vi "Camera.vi"() -> ()   [LabVIEW 2016]
uses:
  <vilib>/rvi/Emulation/niFpgaGetClockAttributes.vi
  <vilib>/rvi/Emulation/niFpgaSctlEmulationGetInTimedLoop.vi
  <vilib>/rvi/Emulation/niFpgaEmulationReportErrorSimple.vi
  <vilib>/rvi/eio/common/nirviEmuTemplateMethod_errors.vi
  <vilib>/rvi/Emulation/niFpgaCriticalErrorInLSC.vi
  <vilib>/eio/EIONode/EIONode.xnode
panel:
  in  "Fly View Frame Rate = R 2":i16=10
  in  "Tlow = t":i16=9
  in  "Arena View Frame Rate = R":i16=200
  out "Camera flash time":i16
  in  "Camera flash time t":i16
  in  "Flash":bool
  # "** Frequency  = 1 / (Fly View R * 0.0001)   i.e R = 10, Frequency = 1000Hz"
  # "**T period = R*100µs,      T low = t*100 µs"
  # "** Frequency  = 1 / (R * 0.0001)   i.e R = 100, Frequency = 100Hz"
  # "** Trigger the fluorenscence camera (Arena View R - x ) *100 microseconds earlier\n      i.e Arena View R = 100, x = 98,\n           offset x = (100 - 98) * 100 µs = 200 µs"
  # "** Camera flash time is set to be the time for triggering the flash at the end of every video.\n** The unit is second."
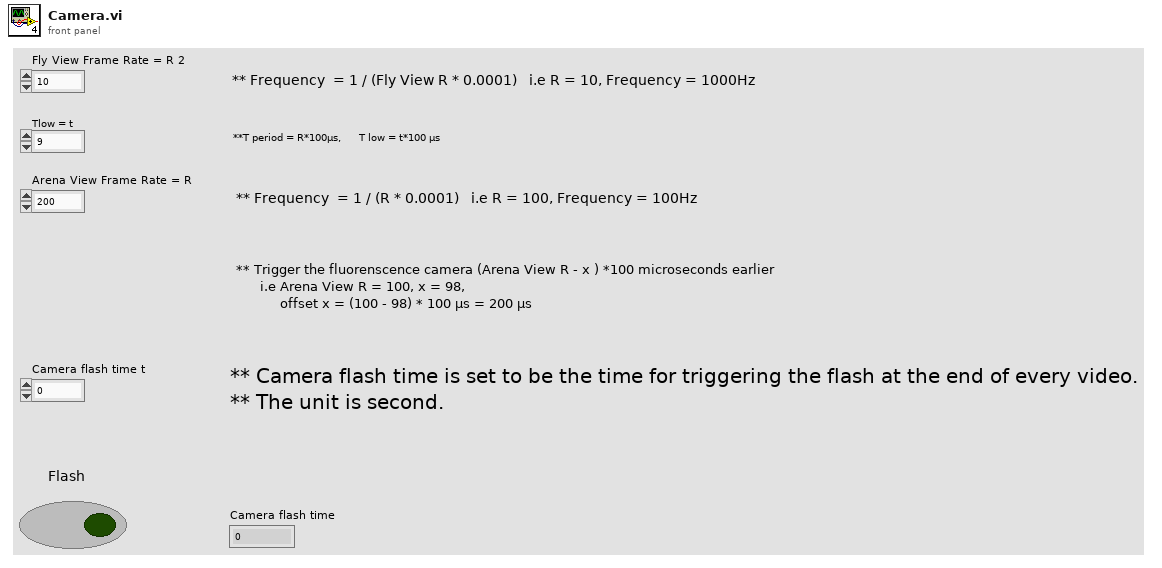
[diagram p1: front panel]
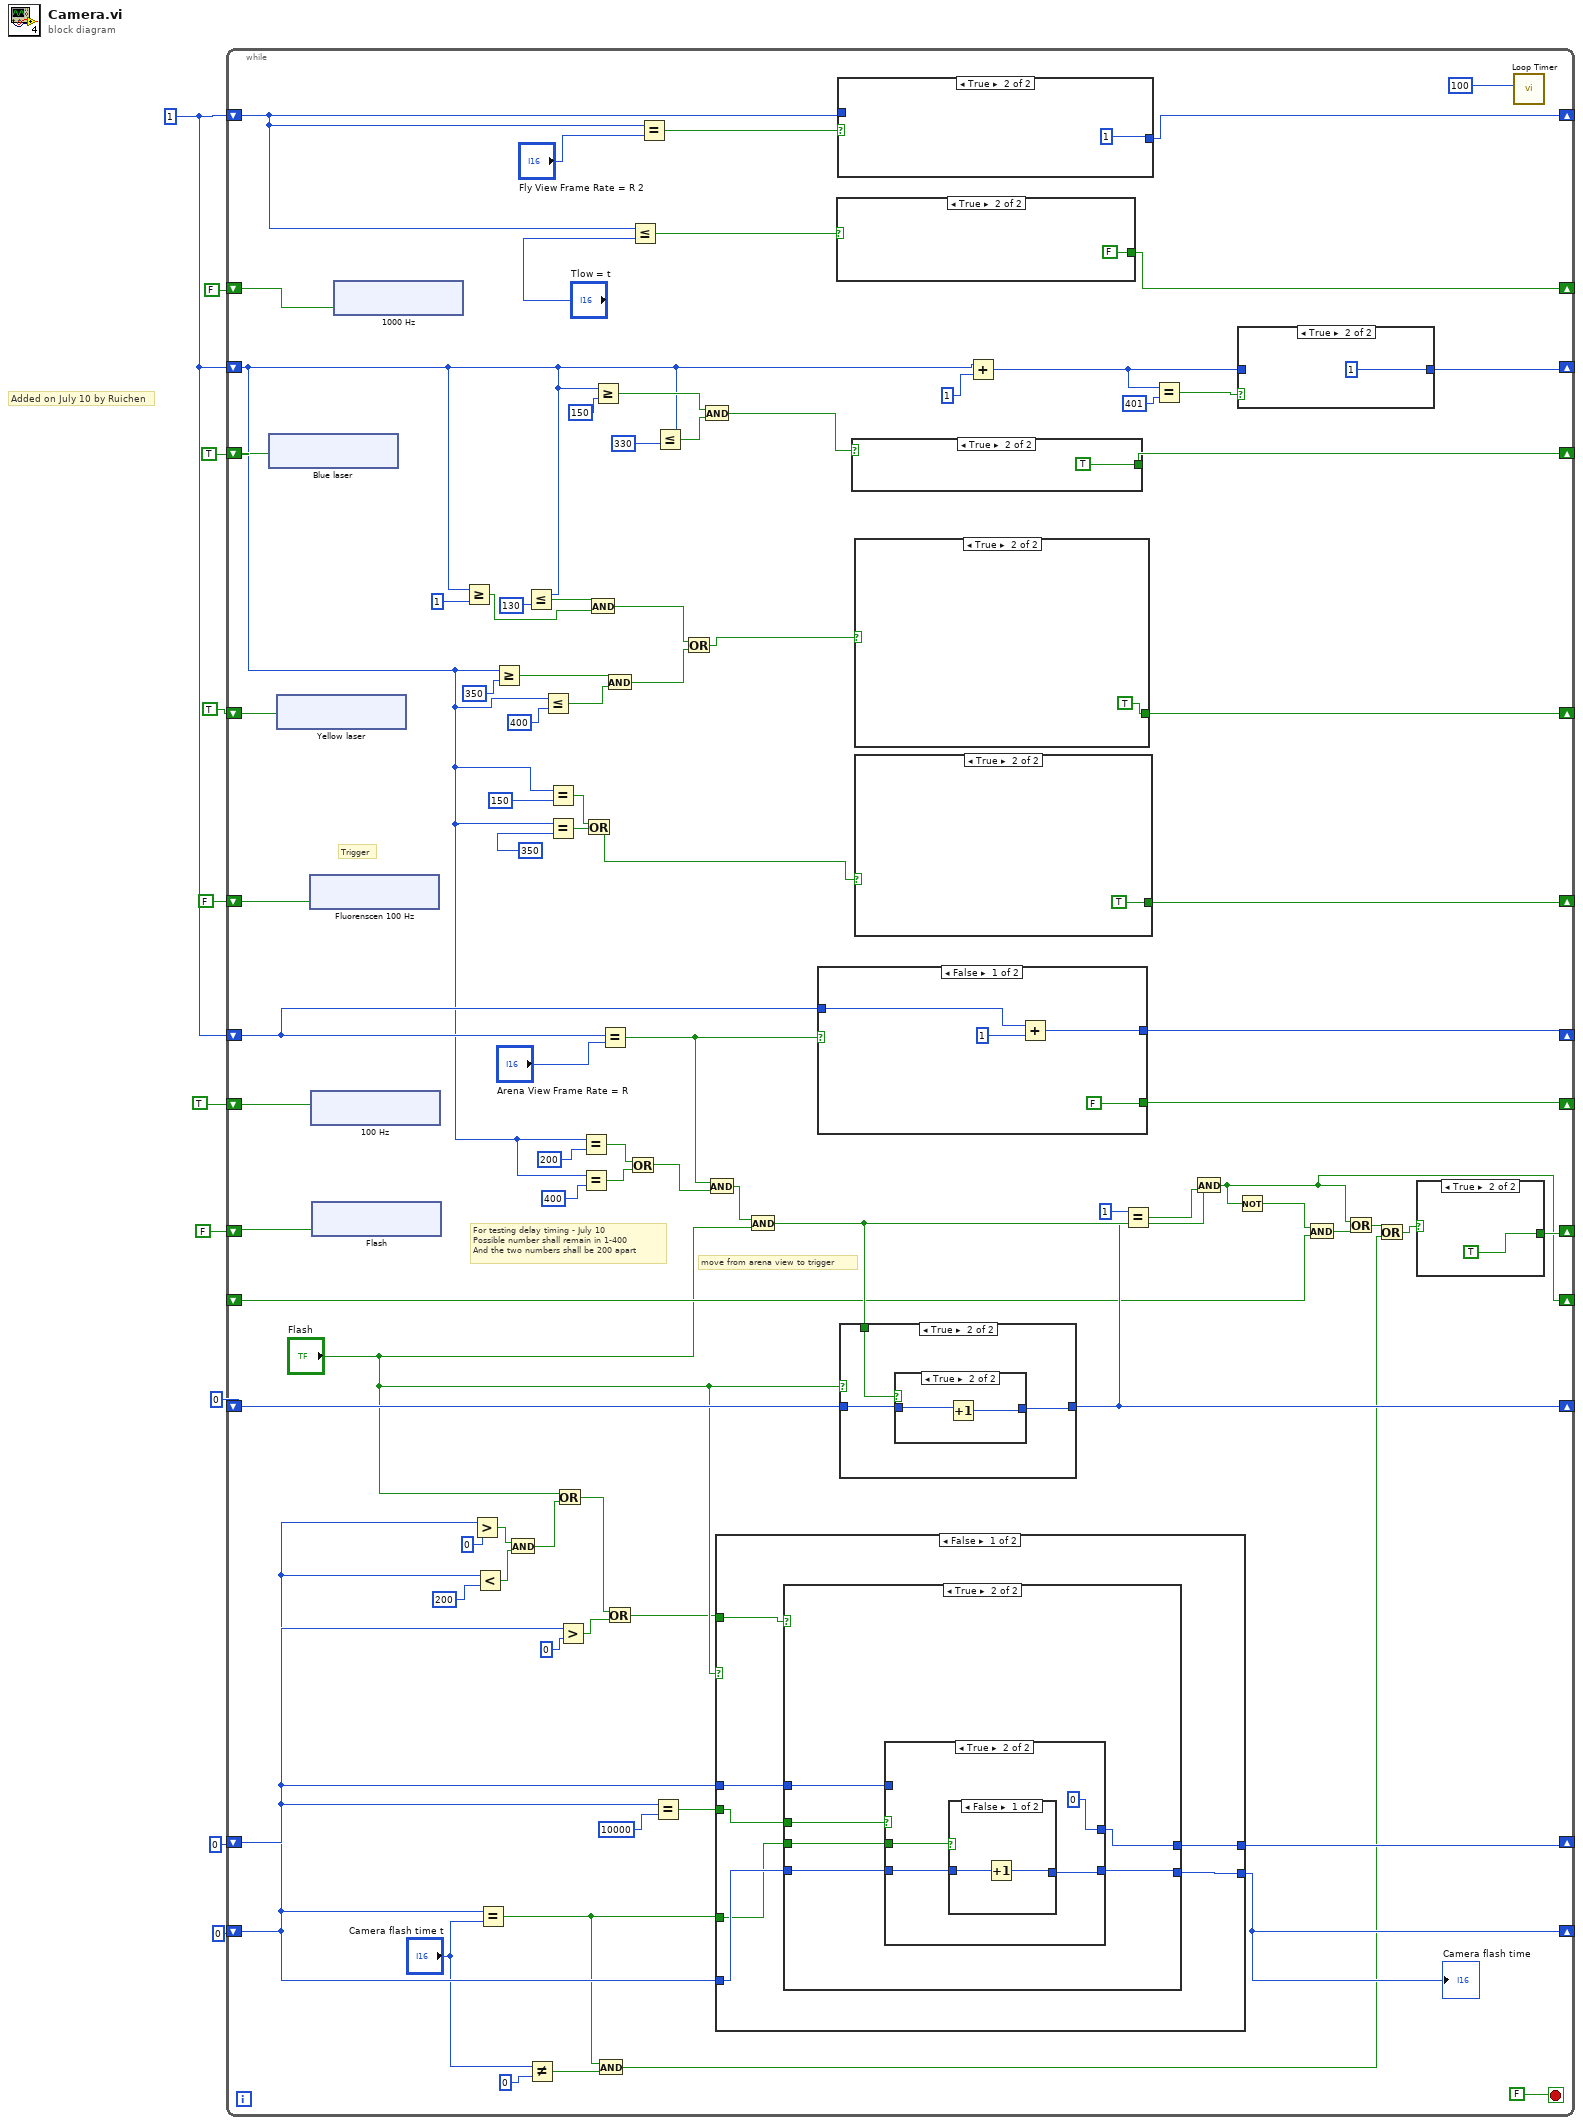
[diagram p0: block diagram]
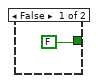
[diagram p2: hidden frame]
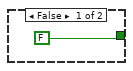
[diagram p4: hidden frame]
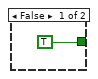
[diagram p5: hidden frame]
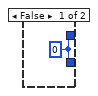
[diagram p6: hidden frame]
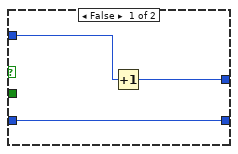
[diagram p7: hidden frame]
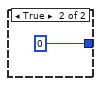
[diagram p8: hidden frame]
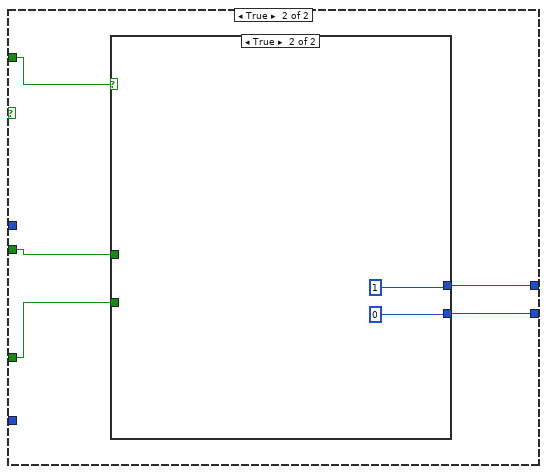
[diagram p9: hidden frame]
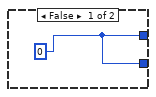
[diagram p10: hidden frame]
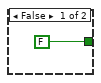
[diagram p11: hidden frame]
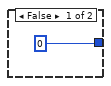
[diagram p12: hidden frame]
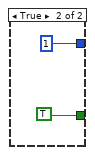
[diagram p14: hidden frame]
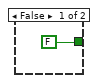
[diagram p15: hidden frame]
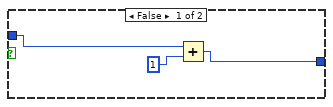
[diagram p16: hidden frame]
diagram:
  w1 = i16 1
  # "Added on July 10 by Ruichen"
  n1 = while {
    shift-right: [w54] -> _
    shift-left: FALSE -> [w99]
    shift-right: [w97] -> _
    shift-left: w1 -> [w51]
    shift-right: [w95] -> _
    shift-left: FALSE -> [w96]
    shift-right: [w94] -> _
    shift-left: TRUE -> [w90]
    shift-right: [w93] -> _
    shift-left: w1 -> [w85]
    shift-right: [w87] -> _
    shift-left: i16 0 -> [w91]
    shift-right: [w83] -> _
    shift-left: FALSE -> [w84]
    shift-right: [w79] -> _
    shift-left: _ -> [w80]
    shift-right: [w73] -> _
    shift-left: i16 0 -> [w66]
    shift-right: [w74] -> _
    shift-left: i16 0 -> [w60]
    shift-right: [w46] -> _
    shift-left: w1 -> [w12]
    shift-right: [w49] -> _
    shift-left: TRUE -> [w50]
    shift-right: [w44] -> _
    shift-left: TRUE -> [w45]
    stop <- FALSE stop-if-true
    # "For testing delay timing - July 10\nPossible number shall remain in 1-400\nAnd the two numbers shall be 200 apart"
    # "move from arena view to trigger"
    # "Trigger"
    n2 = xnode "Blue laser"("ConnectorC/DIO4"=w50) -> ()  [unwired: 1 in, 1 out]
    n3 = xnode "Yellow laser"("ConnectorC/DIO5"=w45) -> ()  [unwired: 1 in, 1 out]
    n4 = xnode "Fluorenscen 100 Hz"("ConnectorC/DIO1"=w96) -> ()  [unwired: 1 in, 1 out]
    n5 = xnode "100 Hz"("ConnectorC/DIO2"=w90) -> ()  [unwired: 1 in, 1 out]
    n6 = xnode "Flash"("ConnectorC/DIO3"=w84) -> ()  [unwired: 1 in, 1 out]
    n7 = xnode "1000 Hz"("ConnectorC/DIO0"=w99) -> ()  [unwired: 1 in, 1 out]
    n8 = Greater Or Equal?(x=w12, y=i16 1) -> (x >= y?=w30:bool)
    n9 = Greater?(x=w60, y=i16 0) -> (0:w63:bool)
    n10 = Less?(x=w60, y=i16 200) -> (x < y?=w62:bool)
    n11 = Equal?(x=w60, y="Camera flash time t") -> (x = y?=w56:bool)
    n12 = Greater Or Equal?(x=w12, y=i16 350) -> (x >= y?=w33:bool)
    n13 = And(x=w63, y=w62) -> (x .and. y?=w61:bool)
    n14 = Less Or Equal?(x=w12, y=i16 130) -> (x <= y?=w31:bool)
    n15 = Not Equal?(x="Camera flash time t", y=i16 0) -> (x != y?=w57:bool)
    n16 = Less Or Equal?(x=w12, y=i16 400) -> (x <= y?=w34:bool)
    n17 = Equal?(x=w12, y=i16 150) -> (x = y?=w42:bool)
    n18 = Equal?(x=w12, y=i16 350) -> (x = y?=w40:bool)
    n19 = Or(x="Flash", y=w61) -> (x .or. y?=w68:bool)
    n20 = Greater?(x=w66, y=i16 0) -> (0:w69:bool)
    n21 = Equal?(x=w12, y=i16 200) -> (x = y?=w20:bool)
    n22 = Equal?(x=w12, y=i16 400) -> (x = y?=w19:bool)
    n23 = Or(x=w42, y=w40) -> (x .or. y?=w23:bool)
    n24 = And(x=w31, y=w30) -> (x .and. y?=w29:bool)
    n25 = Greater Or Equal?(x=w12, y=i16 150) -> (x >= y?=w26:bool)
    n26 = And(x=w56, y=w57) -> (x .and. y?=w55:bool)
    n27 = Equal?(x=w85, y="Arena View Frame Rate = R") -> (x = y?=w18:bool)
    n28 = And(x=w33, y=w34) -> (x .and. y?=w32:bool)
    n29 = Or(x=w68, y=w69) -> (x .or. y?=w67:bool)
    n30 = Or(x=w20, y=w19) -> (x .or. y?=w17:bool)
    n31 = Less Or Equal?(x=w51, y="Tlow = t") -> (x <= y?=w53:bool)
    n32 = Equal?(x=w51, y="Fly View Frame Rate = R 2") -> (x = y?=w92:bool)
    n33 = Equal?(x=w66, y=i16 10000) -> (x = y?=w72:bool)
    n34 = Less Or Equal?(x=w12, y=i16 330) -> (x <= y?=w25:bool)
    n35 = Or(x=w29, y=w32) -> (x .or. y?=w39:bool)
    n36 = And(x=w26, y=w25) -> (x .and. y?=w24:bool)
    n37 = And(x=w18, y=w17) -> (x .and. y?=w16:bool)
    n38 = case shown="False" "Flash" {
      tunnel: [w113 w136] -> w74
      tunnel: [w114 w135] -> w73
      tunnel: w66 -> [w111 _]
      tunnel: w72 -> [w112 w134]
      tunnel: w56 -> [w108 w133]
      tunnel: w60 -> [w110 _]
      tunnel: w67 -> [w109 w132]
      frame False {
        n39 = case shown="True" w109 {
          tunnel: [w115 w119] -> w114
          tunnel: [w115 w118] -> w113
          tunnel: w112 -> [_ w121]
          tunnel: w111 -> [_ w120]
          tunnel: w110 -> [_ w117]
          tunnel: w108 -> [_ w116]
          frame False {
            w115 = i16 0
          }
          frame True {
            n40 = case shown="True" w121 {
              tunnel: w120 -> [w124 _]
              tunnel: [w123 i16 0] -> w119
              tunnel: [w122 w127] -> w118
              tunnel: w117 -> [w122 w126]
              tunnel: w116 -> [_ w125]
              frame False {
                n41 = Increment(x=w124) -> (x+1=w123:i16)
              }
              frame True {
                n42 = case shown="False" w125 {
                  tunnel: [w129 i16 0] -> w127
                  tunnel: w126 -> [w130 _]
                  frame False {
                    n43 = Increment(x=w130) -> (x+1=w129:i16)
                  }
                  frame True {
                  }
                }
              }
            }
          }
        }
      }
      frame True {
        n44 = case shown="True" w132 {
          tunnel: [w137 i16 1] -> w135
          tunnel: w133 -> [_ _]
          tunnel: [w137 i16 0] -> w136
          tunnel: w134 -> [_ _]
          frame False {
            w137 = i16 0
          }
          frame True {
          }
        }
      }
    }
    "Camera flash time" <- w74
    n45 = And(x=w16, y="Flash") -> (x .and. y?=w89:bool)
    n46 = case shown="False" w18 {
      tunnel: [FALSE TRUE] -> w94
      tunnel: [w150 i16 1] -> w93
      tunnel: w85 -> [w152 _]
      frame False {
        n47 = Add(x=w152, y=i16 1) -> (x+y=w150:i16)
      }
      frame True {
      }
    }
    n48 = case shown="True" w53 {
      tunnel: [TRUE FALSE] -> w54
      frame False {
      }
      frame True {
      }
    }
    n49 = case shown="True" w92 {
      tunnel: [w158 i16 1] -> w97
      tunnel: w51 -> [w157 _]
      frame False {
        n50 = Add(x=w157, y=i16 1) -> (x+y=w158:i16)
      }
      frame True {
      }
    }
    n51 = case shown="True" "Flash" {
      tunnel: w91 -> [_ w144]
      tunnel: [i16 0 w143] -> w87
      tunnel: w89 -> [_ w145]
      frame False {
      }
      frame True {
        n52 = case shown="True" w145 {
          tunnel: w144 -> [w146 w148]
          tunnel: [w146 w147] -> w143
          frame False {
          }
          frame True {
            n53 = Increment(x=w148) -> (x+1=w147:i16)
          }
        }
      }
    }
    n54 = case shown="True" w24 {
      tunnel: [FALSE TRUE] -> w49
      frame False {
      }
      frame True {
      }
    }
    n55 = case shown="True" w39 {
      tunnel: [FALSE TRUE] -> w44
      frame False {
      }
      frame True {
      }
    }
    n56 = case shown="True" w23 {
      tunnel: [FALSE TRUE] -> w95
      frame False {
      }
      frame True {
      }
    }
    n57 = Add(x=w12, y=i16 1) -> (x+y=w11:i16)
    n58 = Equal?(x=i16 1, y=w87) -> (x = y?=w86:bool)
    n59 = Equal?(x=w11, y=i16 401) -> (x = y?=w47:bool)
    n60 = And(x=w89, y=w86) -> (x .and. y?=w79:bool)
    n61 = Not(x=w79) -> (.not. x?=w81:bool)
    n62 = case shown="True" w47 {
      tunnel: [w102 i16 1] -> w46
      tunnel: w11 -> [w102 _]
      frame False {
      }
      frame True {
      }
    }
    n63 = And(x=w81, y=w80) -> (x .and. y?=w82:bool)
    n64 = Or(x=w79, y=w82) -> (x .or. y?=w77:bool)
    n65 = Or(x=w77, y=w55) -> (x .or. y?=w76:bool)
    n66 = case shown="True" w76 {
      tunnel: [FALSE TRUE] -> w83
      frame False {
      }
      frame True {
      }
    }
    n67 = call "Loop Timer"("Count(uSec)"=u32 100) -> ()  [unwired: 1 out]
  }
